vi "http tls handle content data.vi"(6 "exec queue":refnum<queue>, 7 "buffer in":string, 9 "server properties":T1={"max url size"=8000, "max header"=8000, "timeout ms"=5000, "max data size"=104857600}, 10 "application request":T2, 11 "lvlibretls connection in":refnum<class "lvlibretls connection.lvclass">) -> (3 "abort":bool, 5 "buffer out":string)   [LabVIEW 2016]
uses:
  HTTP server/http request.ctl
  HTTP server/http method.ctl
  HTTP headers/http header data.ctl
  HTTP server/http server properties.ctl
  lvlibtls/socket connection/lvlibretls connection.lvclass
  HTTP server/http chunked encoding state.ctl
  <vilib>/dlg_ctls.llb/Space Constant.vi
  HTTP headers/http add header to set.vi
  HTTP server/Basic HTTP server.lvclass
  HTTP headers/http headers.lvlib
  TLS HTTP server.lvclass
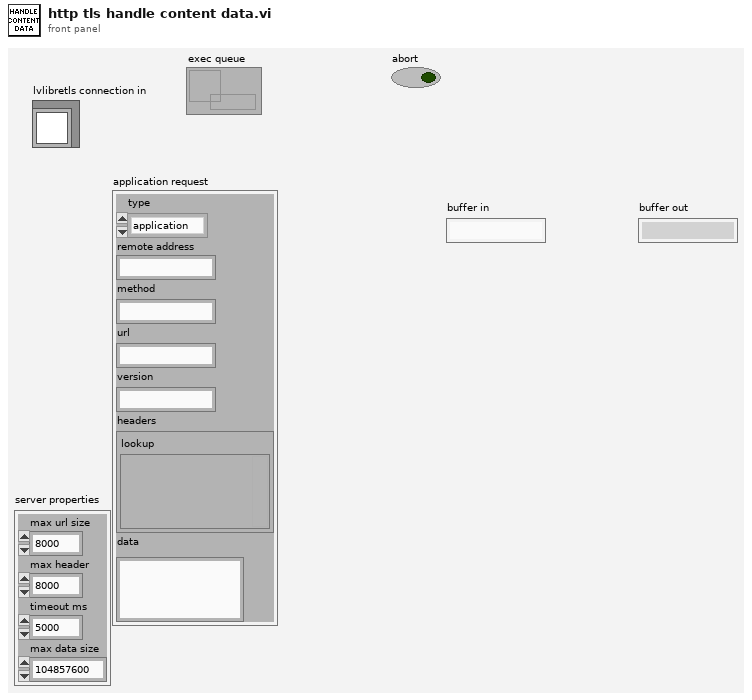
[diagram p1: front panel]
types:
  T1 = typedef "Basic HTTP server.lvclass/http server properties.ctl" = cluster{"max url size":i32, "max header":i32, "timeout ms":i32, "max data size":i32}
  T2 = typedef "Basic HTTP server.lvclass/http request.ctl" = cluster{"type":T3, "remote address":string, "method":string, "url":string, "version":string, "headers":T4, "data":string}
  T3 = typedef "Basic HTTP server.lvclass/http method.ctl" = enum16{"application", "error", "upgrade", "expect"}
  T4 = typedef "http headers.lvlib/http header data.ctl" = cluster{"lookup":variant}
  T5 = typedef "Basic HTTP server.lvclass/http chunked encoding state.ctl" = enum16{"length", "data", "trailer"}
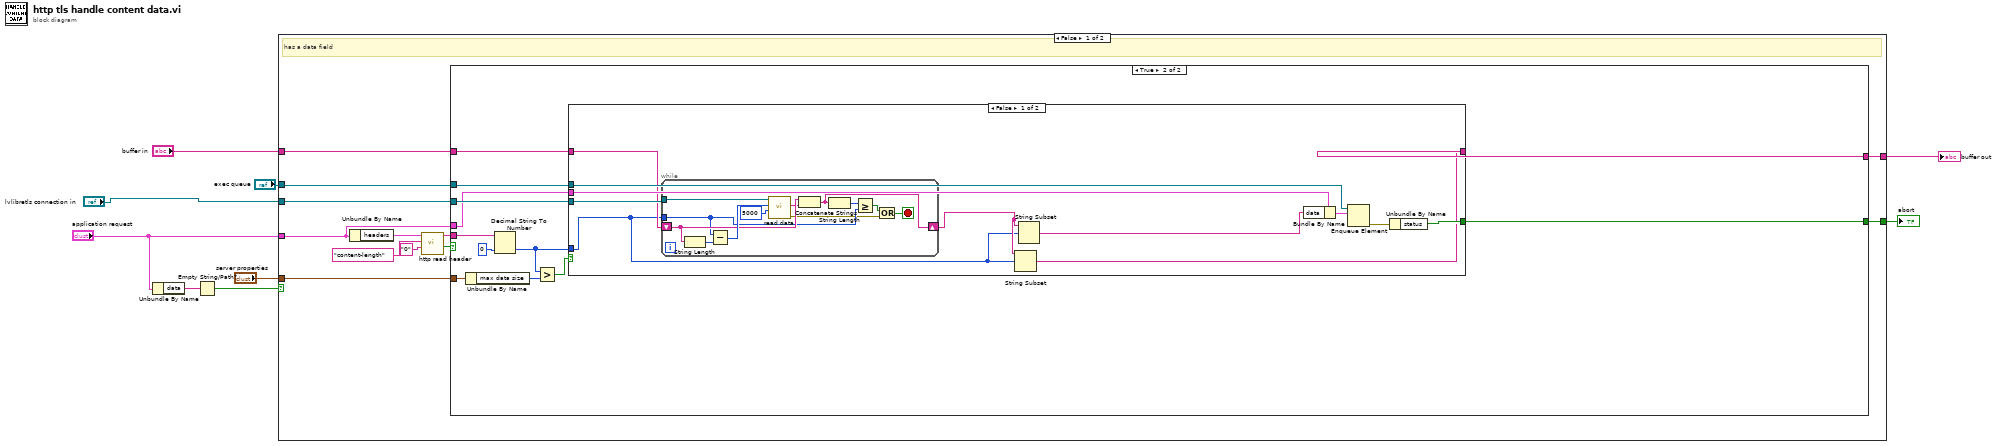
[diagram p0: block diagram]
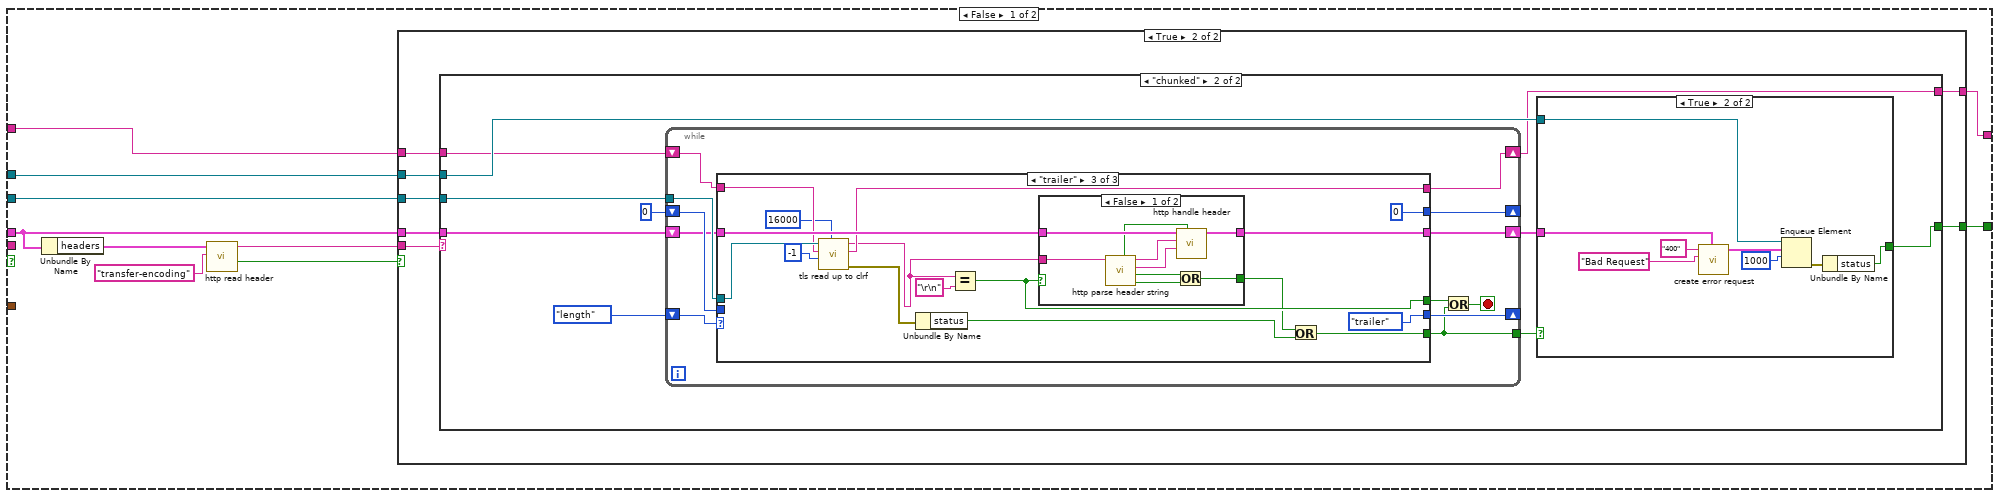
[diagram p2: hidden frame]
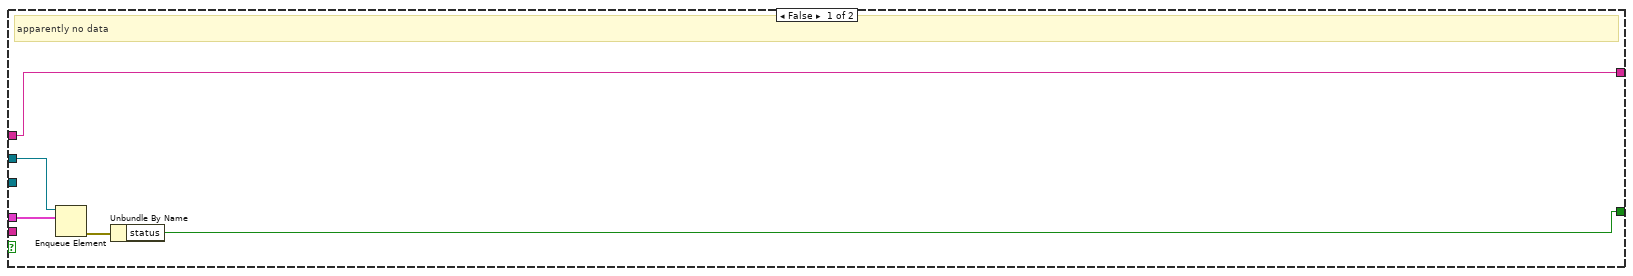
[diagram p3: hidden frame]
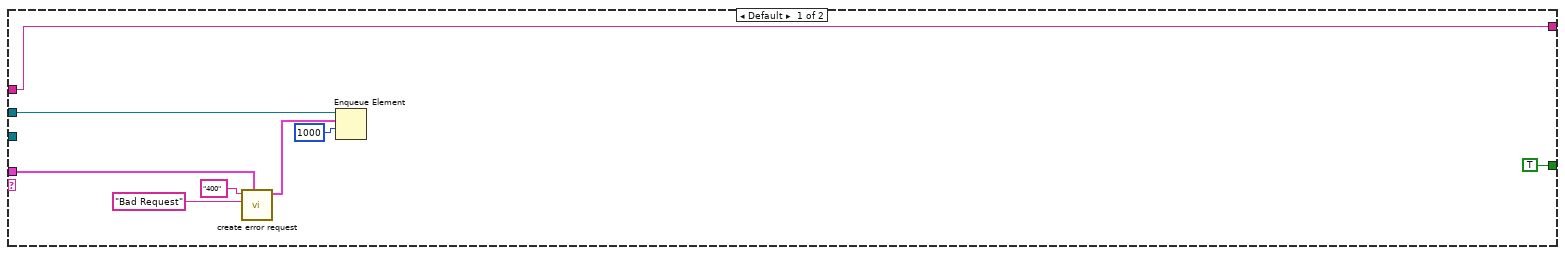
[diagram p4: hidden frame]
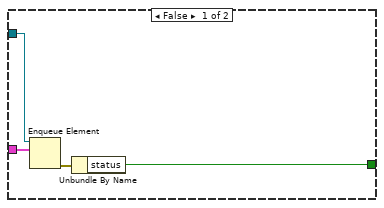
[diagram p5: hidden frame]
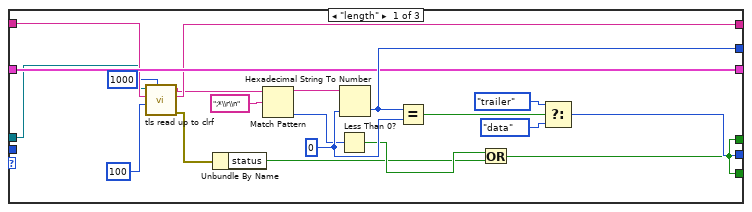
[diagram p6: hidden frame]
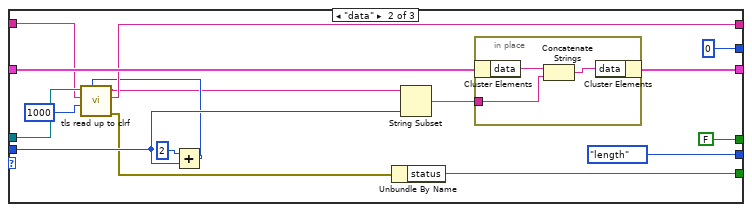
[diagram p7: hidden frame]
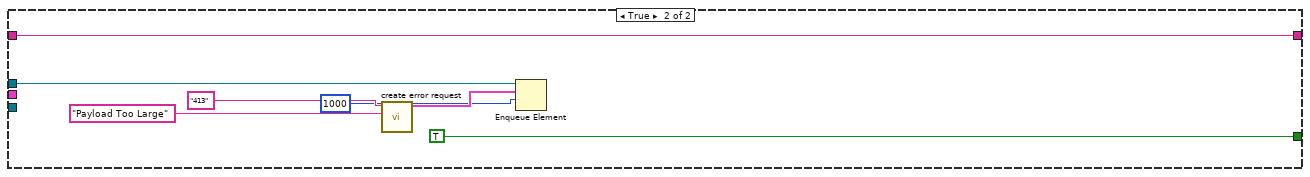
[diagram p9: hidden frame]
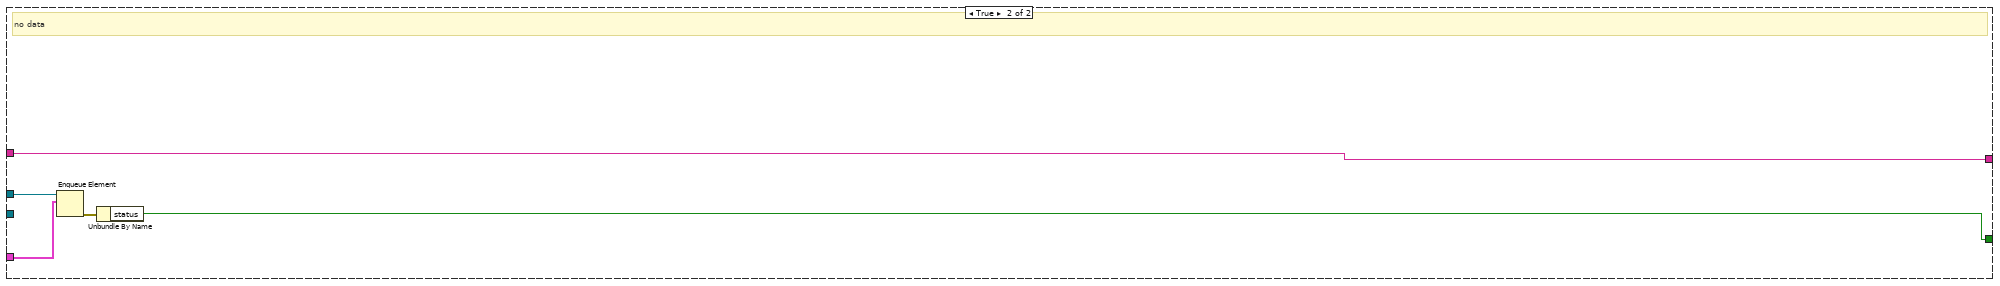
[diagram p10: hidden frame]
diagram:
  n1 = Unbundle By Name("application request") -> ("data"=w5:string)
  n2 = Empty String/Path?(string/path=w5) -> (empty?=w4:bool)
  n3 = case shown="False" w4 {
    tunnel: "lvlibretls connection in" -> [w21 _]
    tunnel: [w20 w194] -> w9
    tunnel: "server properties" -> [w19 _]
    tunnel: "exec queue" -> [w18 w196]
    tunnel: "application request" -> [w17 w197]
    tunnel: [w10 w193] -> w2
    tunnel: "buffer in" -> [w11 w193]
    frame False {
      # "has a data field"
      n4 = Unbundle By Name(w17) -> ("headers"=w16:T4)
      n5 = call "http read header.vi"("default value"="0", "header field name"="content-length" ("name"), "headers"=w16) -> ("found"=w14:bool, "value"=w13:string)  [unwired: 7 in]
      n6 = case shown="True" w14 {
        tunnel: w17 -> [w30 w154]
        tunnel: w21 -> [w29 w161]
        tunnel: [w31 w160] -> w20
        tunnel: w19 -> [_ w159]
        tunnel: w18 -> [w28 w155]
        tunnel: w13 -> [_ w153]
        tunnel: w11 -> [w23 w152]
        tunnel: [w22 w151] -> w10
        frame False {
          n7 = Unbundle By Name(w30) -> ("headers"=w27:T4)
          n8 = call "http read header.vi"("header field name"="transfer-encoding" ("name"), "headers"=w27) -> ("found"=w25:bool, "value"=w24:string)  [unwired: 8 in]
          n9 = case shown="True" w25 {
            tunnel: [w33 w43] -> w31
            tunnel: w30 -> [w36 w40]
            tunnel: w29 -> [_ w42]
            tunnel: w28 -> [w35 w41]
            tunnel: w24 -> [_ w39]
            tunnel: w23 -> [w32 w38]
            tunnel: [w32 w37] -> w22
            frame False {
              # "apparently no data"
              n10 = Enqueue Element(queue=w35, element=w36) -> (error out=w34:errorcluster)  [unwired: 2 in, 2 out]
              n11 = Unbundle By Name(w34) -> ("status"=w33:bool)
            }
            frame True {
              n12 = case shown="\"chunked\"" w39 {
                tunnel: [TRUE w54] -> w43
                tunnel: w40 -> [w45 w58]
                tunnel: w42 -> [_ w60]
                tunnel: w41 -> [w46 w55]
                tunnel: w38 -> [w44 w53]
                tunnel: [w44 w52] -> w37
                frame Default {
                  n13 = call "create error request.vi"("incoming request"=w45, "reason"="Bad Request" ("status string"), "code"="400") -> ("element"=w48:T2)  [unwired: 8 in]
                  n14 = Enqueue Element(queue=w46, element=w48, timeout in ms (-1)=1000) -> ()  [unwired: 1 in, 3 out]
                }
                frame "chunked" {
                  n15 = while {
                    shift-right: [w83] -> _
                    shift-left: http_chunked_encoding_state."length" -> [w85]
                    tunnel: w60 -> [w84]
                    shift-right: [w81] -> _
                    shift-left: 0 ("default (0 I32)") -> [w80]
                    shift-right: [w78] -> w56
                    shift-left: w58 -> [w79]
                    tunnel: [w76] -> w57
                    shift-right: [w74] -> w52
                    shift-left: w53 -> [w75]
                    stop <- w77 stop-if-true
                    n16 = case shown="\"trailer\"" w85 {
                      tunnel: w84 -> [w87 w112 w131]
                      tunnel: [w97 http_chunked_encoding_state."length" http_chunked_encoding_state."trailer"] -> w83
                      tunnel: [w94 FALSE w136] -> w82
                      tunnel: [w102 0 0] -> w81
                      tunnel: w80 -> [_ w120 _]
                      tunnel: w79 -> [w96 w114 w134]
                      tunnel: [w96 w113 w135] -> w78
                      tunnel: [w94 w115 w133] -> w76
                      tunnel: w75 -> [w92 w111 w130]
                      tunnel: [w91 w110 w129] -> w74
                      frame "length" {
                        w103 = 0 ("default (0 I32)")
                        n17 = call "tls read up to clrf.vi"("max size"=1000 ("bytes to read"), "timeout ms"=100 ("timeout ms (25000)"), "buffer in"=w92, "lvlibretls connection in"=w87) -> ("error out"=w89:errorcluster, "buffer out"=w91:string, "line out"=w90:string)  [unwired: 5 in]
                        n18 = Unbundle By Name(w89) -> ("status"=w93:bool)
                        n19 = Match Pattern(string=w90, regular expression=";*\\r\\n") -> (before substring=w104:string, offset past match=w101:i32)  [unwired: 1 in, 2 out]
                        n20 = Less Than 0?(x=w101) -> (x < 0?=w95:bool)
                        n21 = Hexadecimal String To Number(string=w104, default (0uL)=w103) -> (number=w102:i32)  [unwired: 1 in, 1 out]
                        n22 = Equal?(x=w102, y=w103) -> (x = y?=w100:bool)
                        n23 = Or(x=w95, y=w93) -> (x .or. y?=w94:bool)
                        n24 = Select(t=http_chunked_encoding_state."trailer", s=w100, f=http_chunked_encoding_state."data") -> (s? t:f=w97:T5)
                      }
                      frame "data" {
                        n25 = Add(x=2, y=w120) -> (x+y=w108:i32)
                        n26 = call "tls read up to clrf.vi"("max size"=w108, "timeout ms"=1000 ("timeout ms (25000)"), "buffer in"=w111, "lvlibretls connection in"=w112) -> ("error out"=w106:errorcluster, "buffer out"=w110:string, "line out"=w107:string)  [unwired: 5 in]
                        n27 = Unbundle By Name(w106) -> ("status"=w115:bool)
                        n28 = String Subset(string=w107, length (rest)=w120) -> (substring=w119:string)  [unwired: 1 in]
                        n29 = in-place {
                          in-place-border: w119 -> [w124]
                          n30 = in-place-cluster #1(w114) -> ("data"=w123:string)
                          n31 = Concatenate Strings(w123, w124) -> (w122:string)
                          n32 = in-place-cluster #1("data"=w122) -> (w113:T2)
                        }
                      }
                      frame "trailer" {
                        n33 = call "tls read up to clrf.vi"("max size"=16000 ("bytes to read"), "timeout ms"=-1 ("timeout ms (25000)"), "buffer in"=w130, "lvlibretls connection in"=w131) -> ("error out"=w127:errorcluster, "buffer out"=w129:string, "line out"=w128:string)  [unwired: 5 in]
                        n34 = Unbundle By Name(w127) -> ("status"=w139:bool)
                        n35 = Equal?(x=w128, y="\r\n" ("x")) -> (x = y?=w136:bool)
                        n36 = case shown="False" w136 {
                          tunnel: [w149 w150] -> w135
                          tunnel: w134 -> [w148 w150]
                          tunnel: [w144 _] -> w132
                          tunnel: w128 -> [w145 _]
                          frame False {
                            n37 = call "http parse header string.vi"("raw string"=w145) -> ("no field name"=w143:bool, "no crlf"=w147:bool, "header field data"=w146:string, "header field name"=w142:string, "continuation"=w141:bool)  [unwired: 6 in]
                            n38 = Or(x=w147, y=w143) -> (x .or. y?=w144:bool)
                            n39 = call "http handle header.vi"("continuation"=w141, "header field data"=w146, "header field name"=w142, "application request in"=w148) -> ("application request out"=w149:T2)  [unwired: 7 in]
                          }
                          frame True {
                          }
                        }
                        n40 = Or(x=w132, y=w139) -> (x .or. y?=w133:bool)
                      }
                    }
                    n41 = Or(x=w82, y=w76) -> (x .or. y?=w77:bool)
                  }
                  n42 = case shown="True" w57 {
                    tunnel: w56 -> [w64 w67]
                    tunnel: w55 -> [w65 w68]
                    tunnel: [w62 w73] -> w54
                    frame False {
                      n43 = Enqueue Element(queue=w65, element=w64) -> (error out=w63:errorcluster)  [unwired: 2 in, 2 out]
                      n44 = Unbundle By Name(w63) -> ("status"=w62:bool)
                    }
                    frame True {
                      n45 = call "create error request.vi"("incoming request"=w67, "reason"="Bad Request" ("status string"), "code"="400") -> ("element"=w71:T2)  [unwired: 8 in]
                      n46 = Enqueue Element(queue=w68, element=w71, timeout in ms (-1)=1000) -> (error out=w66:errorcluster)  [unwired: 1 in, 2 out]
                      n47 = Unbundle By Name(w66) -> ("status"=w73:bool)
                    }
                  }
                }
              }
            }
          }
        }
        frame True {
          n48 = Unbundle By Name(w159) -> ("max data size"=w158:i32)
          n49 = Decimal String To Number(string=w153, default (0L)=0 ("default (0 I32)")) -> (number=w157:i32)  [unwired: 1 in, 1 out]
          n50 = Greater?(x=w157, y=w158) -> (0:w156:bool)
          n51 = case shown="False" w156 {
            tunnel: w161 -> [w168 _]
            tunnel: [w173 TRUE ("status")] -> w160
            tunnel: w154 -> [w172 _]
            tunnel: w157 -> [w165 _]
            tunnel: w155 -> [w170 w189]
            tunnel: w152 -> [w167 w186]
            tunnel: [w164 w186] -> w151
            frame False {
              n52 = while {
                tunnel: w168 -> [w185]
                shift-right: [w177] -> w166
                shift-left: w167 -> [w182]
                tunnel: w165 -> [w180]
                stop <- w176 stop-if-true
                n53 = String Length(string=w182) -> (length=w181:i32)
                n54 = Subtract(x=w180, y=w181) -> (x-y=w183:i32)
                n55 = call "read data.vi"("timeout"=5000, "max size"=w183, "lvlibretls connection in"=w185) -> ("error out"=w174:errorcluster, "data"=w179:string)  [unwired: 6 in, 1 out]
                n56 = Concatenate Strings(w182, w179) -> (w177:string)
                n57 = String Length(string=w177) -> (length=w178:i32)
                n58 = Greater Or Equal?(x=w178, y=w180) -> (x >= y?=w175:bool)
                n59 = Or(x=w175, y=w174) -> (x .or. y?=w176:bool)
              }
              n60 = String Subset(string=w166, offset (0)=w165) -> (substring=w164:string)  [unwired: 1 in]
              n61 = String Subset(string=w166, offset (0)=w165) -> (substring=w163:string)  [unwired: 1 in]
              n62 = Bundle By Name(cluster=w172, "data"=w163) -> (w169:T2)
              n63 = Enqueue Element(queue=w170, element=w169) -> (error out=w171:errorcluster)  [unwired: 2 in, 2 out]
              n64 = Unbundle By Name(w171) -> ("status"=w173:bool)
            }
            frame True {
              n65 = call "create error request.vi"("reason"="Payload Too Large" ("status string"), "code"="413") -> ("element"=w188:T2)  [unwired: 9 in]
              n66 = Enqueue Element(queue=w189, element=w188, timeout in ms (-1)=1000) -> ()  [unwired: 1 in, 3 out]
            }
          }
        }
      }
    }
    frame True {
      # "no data"
      n67 = Enqueue Element(queue=w196, element=w197) -> (error out=w195:errorcluster)  [unwired: 2 in, 2 out]
      n68 = Unbundle By Name(w195) -> ("status"=w194:bool)
    }
  }
  "abort" <- w9
  "buffer out" <- w2
